vi "global_error_anywhere.vi"() -> ()   [LabVIEW 2011]
panel:
  in  "error anywhere":errorcluster
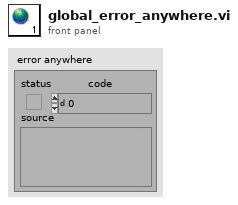
[diagram p1: front panel]
diagram:
